vi "Configure Setpoint Temperature.vi"(8 "error in (no error)":errorcluster, 9 "Setpoint (0)":dbl, 11 "VISA resource name":refnum<visa-resource-name>) -> (0 "error out":errorcluster, 3 "VISA resource name out":refnum<visa-resource-name>)   [LabVIEW 2012, in "Temptronic TP04300.lvlib"]
doc: "This VI configures setpoint temperature.\n\n<b>Setpoint temperature</b>\nValid Range: \n -150.0 to 225.0 in the Cycle Screen for any setpoint\n 25.0 to 225.0 for setpoint #0 in Operator Screen\n 15.0 to 35.0 for setpoint #1 in Operator Screen\n -150.0 to 25.0 for setpoint #2 in Operator Screen\n\nNote: Entering a value greater than maximum air temperature limit or\nless than minimum air temperature limit will cause \"out of range error\""
uses:
  <instrlib>/Temptronic TP04300/Temptronic TP04300.lvlib
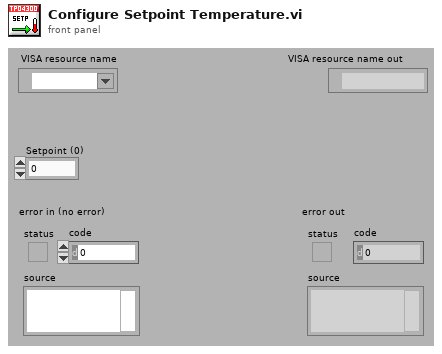
[diagram p1: front panel]
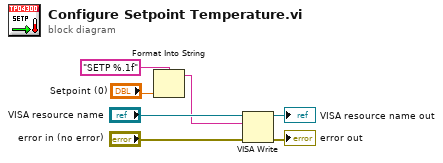
[diagram p0: block diagram]
diagram:
  n1 = Format Into String(format string="SETP %.1f" ("multi-line string"), "Setpoint (0)") -> (resulting string=w3:string)  [unwired: 2 in, 1 out]
  n2 = VISA Write(VISA resource name="VISA resource name", write buffer=w3, error in (no error)="error in (no error)") -> (VISA resource name out=→"VISA resource name out":refnum<visa-resource-name>, error out=→"error out":errorcluster)  [unwired: 1 out]
